vi "CRYGet Window Subpanel Reference.vi"(10 "Sub Panel Name":string="Basic", 11 "VI Ref In":refnum<vi>) -> (1 "SubPnl Refnum":refnum<vi>, 2 "YesNo":bool, 3 "VI Ref Out":refnum<vi>)   [LabVIEW 2013]
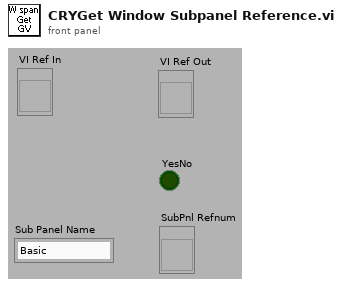
[diagram p1: front panel]
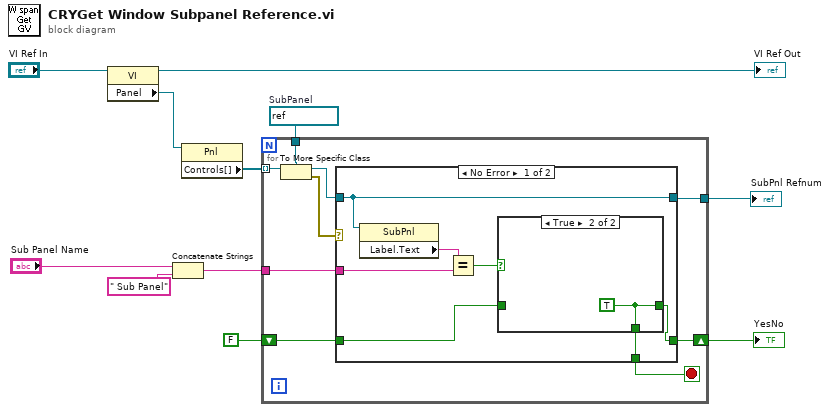
[diagram p0: block diagram]
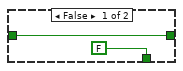
[diagram p2: hidden frame]
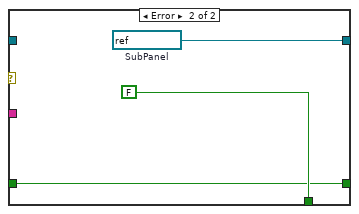
[diagram p3: hidden frame]
diagram:
  w4 = refnum<vi> refnum  # SubPanel
  n1 = property class="VI"(reference="VI Ref In") -> (reference out=→"VI Ref Out":refnum<vi>, "Panel"=w6:refnum<vi>)  [unwired: 1 in, 1 out]
  n2 = Concatenate Strings("Sub Panel Name", " Sub Panel" ("string")) -> (w2:string)
  n3 = property class="Pnl"(reference=w6) -> ("Controls[]"=w5:refnum<vi>[])  [unwired: 1 in, 2 out]
  n4 = for {
    tunnel: w5 -> [w20] mode=indexing
    tunnel: w4 -> [w19]
    tunnel: [w16] -> w11
    tunnel: w2 -> [w14]
    shift-right: [w13] -> w7
    shift-left: FALSE ("Boolean") -> [w12]
    stop <- w15 stop-if-true
    n5 = To More Specific Class(target class=w19, reference=w20) -> (specific class reference=w17:refnum<vi>, error out=w18:errorcluster)  [unwired: 1 in]
    n6 = case shown="No Error" w18 {
      tunnel: w17 -> [w25 _]
      tunnel: [w25 w32] -> w16
      tunnel: [w27 FALSE] -> w15
      tunnel: w14 -> [w23 _]
      tunnel: w12 -> [w22 w31]
      tunnel: [w21 w31] -> w13
      frame No Error {
        n7 = property class="SubPnl"(reference=w25) -> ("Label.Text"=w26:string)  [unwired: 1 in, 2 out]
        n8 = Equal?(x=w26, y=w23) -> (x = y?=w24:bool)
        n9 = case shown="True" w24 {
          tunnel: [FALSE w30] -> w27
          tunnel: w22 -> [w28 _]
          tunnel: [w28 w30] -> w21
          frame False {
          }
          frame True {
            w30 = TRUE
          }
        }
      }
      frame Error {
        w32 = refnum<vi> refnum  # SubPanel
      }
    }
  }
  "SubPnl Refnum" <- w11
  "YesNo" <- w7
